vi "XYZ Stage-Command acknowledgment module.vi"(8 "error in":errorcluster, 10 "State":T1=enum."Wait for acknowledgment", 11 "Acknowledgement Message in":string) -> (0 "error out":errorcluster, 2 "Timed out while waiting for acknowledgement":bool, 3 "Acknowledgement Message out":string)   [LabVIEW 2017]
doc: "This is the interface module handling all inter-process signaling between the main software and the XYZ stage driver."
uses:
  Typedefs/Command acknowledgment states.ctl
  User Interface/Windows/Position control window/Globals/Pos ctrl window globals.vi
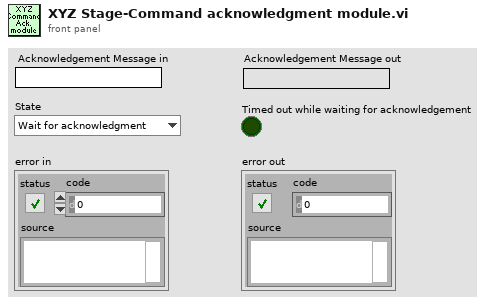
[diagram p1: front panel]
types:
  T1 = typedef "Command acknowledgment states.ctl" = enum16{"Acknowledge", "Wait for acknowledgment", "Release queue"}
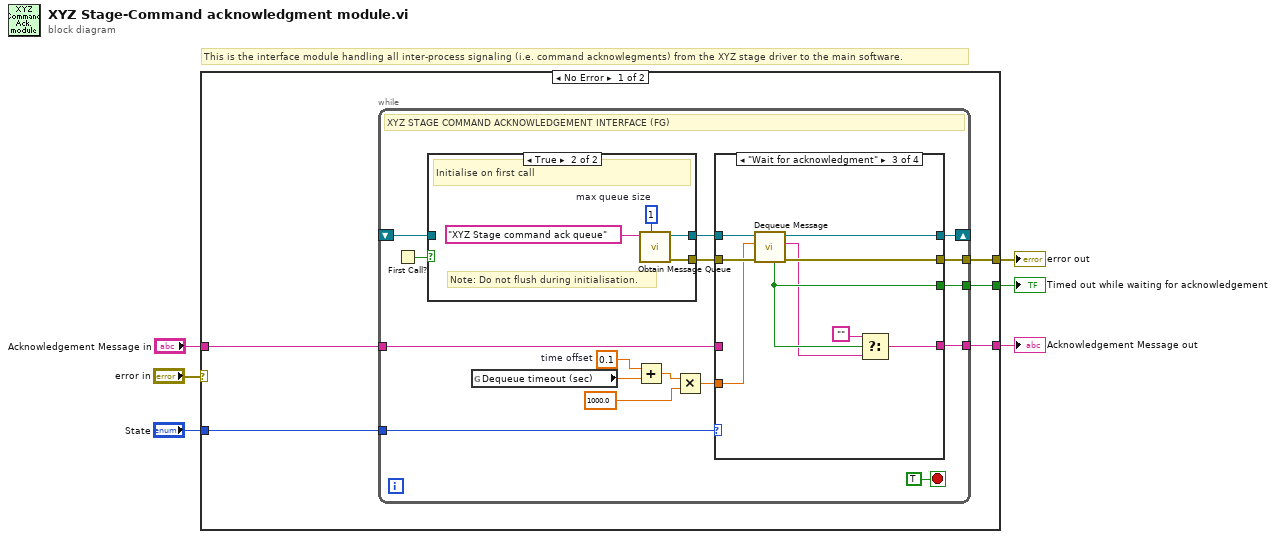
[diagram p0: block diagram]
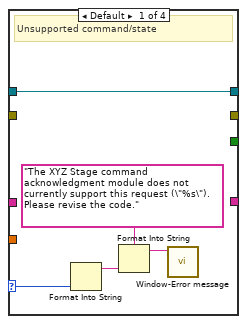
[diagram p2: hidden frame]
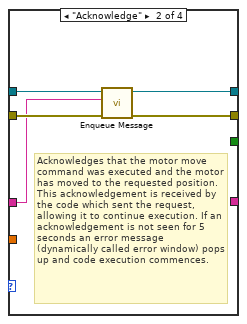
[diagram p3: hidden frame]
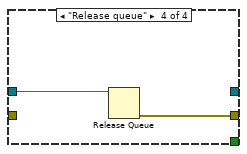
[diagram p4: hidden frame]
diagram:
  # "This is the interface module handling all inter-process signaling (i.e. command acknowlegments) from the XYZ stage driver to the main software."
  n1 = case shown="No Error" "error in" {
    selector: "error in" -> [_ w54]
    tunnel: "State" -> [w9 _]
    tunnel: [w11 _] -> w5
    tunnel: [w10 w54] -> w4
    tunnel: "Acknowledgement Message in" -> [w8 _]
    tunnel: [w7 _] -> w1
    frame No Error {
      n2 = while {
        shift-right: [w23] -> _
        shift-left: _ -> [w25]
        tunnel: w9 -> [w19]
        tunnel: [w22] -> w11
        tunnel: [w20] -> w10
        tunnel: w8 -> [w18]
        tunnel: [w17] -> w7
        stop <- TRUE stop-if-true
        w12 = 0.1  # time offset
        # "XYZ STAGE COMMAND ACKNOWLEDGEMENT INTERFACE (FG)"
        n3 = First Call?() -> (First Call?: T/F=w26:bool)
        n4 = case shown="True" w26 {
          tunnel: [w49 w51] -> w24
          tunnel: w25 -> [w49 _]
          tunnel: [_ w50] -> w21
          frame False {
          }
          frame True {
            w52 = 1  # max queue size
            # "Note: Do not flush during initialisation."
            # "Initialise on first call"
            n5 = call "Obtain Message Queue.vi"("max queue size (-1, unlimited)"=w52, "Queue name"="XYZ Stage command ack queue") -> ("error out"=w50:errorcluster, "Message Queue"=w51:refnum<queue>)  [unwired: 8 in]
          }
        }
        n6 = global read "Pos ctrl window globals.vi" "Dequeue timeout (sec)"() -> (w14:dbl)
        n7 = Add(x=w12, y=w14) -> (x+y=w13:dbl)
        n8 = Multiply(x=w13, y=1000.0) -> (x*y=w15:dbl)
        n9 = case shown="\"Wait for acknowledgment\"" w19 {
          selector: w19 -> [w31 _ _ _]
          tunnel: w24 -> [w32 w37 w46 w48]
          tunnel: [w32 w36 w45 _] -> w23
          tunnel: [_ _ w42 _] -> w22
          tunnel: w21 -> [_ w35 w44 _]
          tunnel: [_ w34 w43 w47] -> w20
          tunnel: w18 -> [_ w33 _ _]
          tunnel: [_ _ w39 _] -> w17
          tunnel: w15 -> [_ _ w38 _]
          frame Default {
            # "Unsupported command/state"
            n10 = Format Into String(w31) -> (resulting string=w29:string)  [unwired: 3 in, 1 out]
            n11 = Format Into String(format string="The XYZ Stage command acknowledgment module does not currently support this request (\"%s\"). Please revise the code.", w29) -> (resulting string=w28:string)  [unwired: 2 in, 1 out]
            n12 = call "Window-Error message.vi"("Message"=w28) -> ()  [unwired: 10 in, 1 out]
          }
          frame "Acknowledge" {
            # "Acknowledges that the motor move command was executed and the motor has moved to the requested position. This acknowledgement is received by the code which sent the request, allowing it to continue execution. If an acknowledgement is not seen for 5 seconds an error message (dynamically called error window) pops up and code execution commences."
            n13 = call "Enqueue Message.vi"("error in (no error)"=w35, "Message"=w33, "Queue"=w37) -> ("error out"=w34:errorcluster, "Queue out"=w36:refnum<queue>)  [unwired: 7 in]
          }
          frame "Wait for acknowledgment" {
            n14 = call "Dequeue Message.vi"("Error In"=w44, "timeout in ms (-1)"=w38, "Message Queue"=w46) -> ("Error Out"=w43:errorcluster, "Message"=w40:string, "dup Message Queue"=w45:refnum<queue>, "timed out?"=w42:bool)  [unwired: 4 in, 1 out]
            n15 = Select(t="" ("Message"), s=w42, f=w40) -> (s? t:f=w39:string)
          }
          frame "Release queue" {
            n16 = Release Queue(queue=w48) -> (error out=w47:errorcluster)  [unwired: 2 in, 2 out]
          }
        }
      }
    }
    frame Error {
    }
  }
  "Timed out while waiting for acknowledgement" <- w5
  "error out" <- w4
  "Acknowledgement Message out" <- w1
